vi "GatherBLTargets.vi"(11 "BL files folder path":path) -> (1 "BL Targets out":T1[](array[typedef]) {"n" min=0.02 max=0.5 step=0.01 format="%.2f"})   [LabVIEW 2016]
uses:
  BLTarget.ctl
  Globals/Constants_global.vi
panel:
  in  "BL Targets Manual":T1[](array[typedef])=[{"Code"="ASCE7 C", "TI Profile (FS)"=[[25.4, 12.0], [25.4, 14.0], [50.8, 13.0], [50.8, 11.0], [25.4, 12.0]], "n"=0.14}, {"Code"="B2", "TI Profile (FS)"=[[15.0, 25.5], [20.0, 24.3], [25.0, 23.5], [30.0, 22.9], [35.0, 22.3], [45.0, 21.5], [55.0, 20.9], [65.0, 20.4], [80.0, 19.7], [100.0, 19.0], [125.0, 18.2], [150.0, 17.6], [200.0, 16.5], [235.0, 15.8], [300.0, 14.7], [360.0, 13.9]], "n"=0.24}, {"Code"="C1", "TI Profile (FS)"=[[76.2, 10.28], [152.4, 8.46]], "n"=0.139}, {"Code"="C2", "TI Profile (FS)"=[[15.0, 16.0], [20.0, 15.6], [25.0, 15.2], [30.0, 14.9], [35.0, 14.7], [45.0, 14.2], [55.0, 13.9], [65.0, 13.5], [80.0, 13.0], [100.0, 12.5], [125.0, 11.9], [150.0, 11.4], [200.0, 10.5], [235.0, 10.0], [300.0, 9.2], [360.0, 8.6]], "n"=0.16000000000000003}, {"Code"="AB1", "TI Profile (FS)"=[[76.2, 29.33], [152.4, 22.56]], "n"=0.292}, {"Code"="D1", "TI Profile (FS)"=[[76.2, 12.115], [152.4, 11.19]], "n"=0.106}, {"Code"="Cat2", "TI Profile (FS)"=[[10.0, 20.7], [16.7, 19.6], [33.3, 18.3], [50.0, 17.6], [66.7, 17.1], [100.0, 16.2], [133.3, 15.6], [166.7, 15.1], [250.0, 14.0], [333.3, 13.1], [500.0, 11.7], [666.7, 10.8], [833.3, 9.8], [1000.0, 9.2], [1333.3, 8.2], [1666.7, 7.4], [3333.3, 7.4]], "n"=0.202}, {"Code"="Cat3", "TI Profile (FS)"=[[10.0, 27.1], [16.7, 27.1], [33.3, 23.9], [50.0, 22.5], [66.7, 21.5], [100.0, 20.3], [133.3, 19.5], [166.7, 18.8], [250.0, 17.6], [333.3, 16.6], [500.0, 15.0], [666.7, 13.9], [833.3, 12.9], [1000.0, 12.1], [1333.3, 10.8], [1666.7, 9.8], [3333.3, 9.8]], "n"=0.202}] {"n" min=0.02 max=0.5 step=0.01 format="%.2f"}
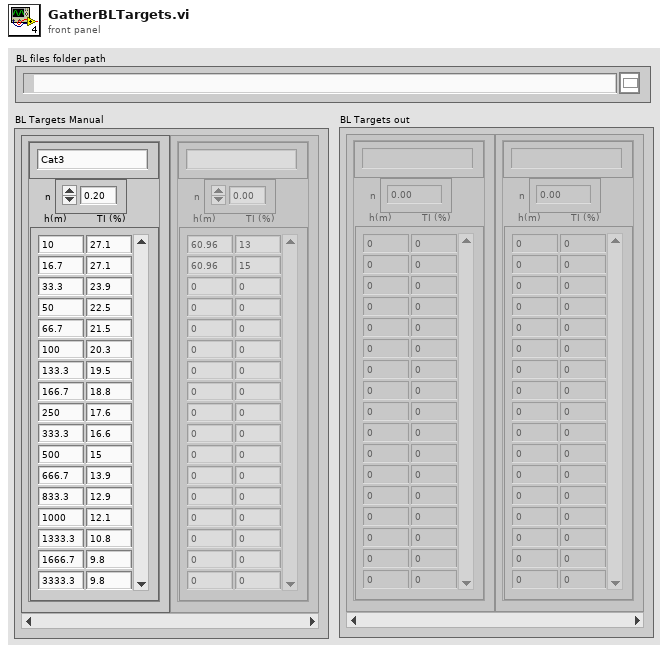
[diagram p1: front panel]
types:
  T1 = typedef "BLTarget.ctl" = cluster{"Code":string, "TI Profile (FS)":dbl[][], "n":dbl}
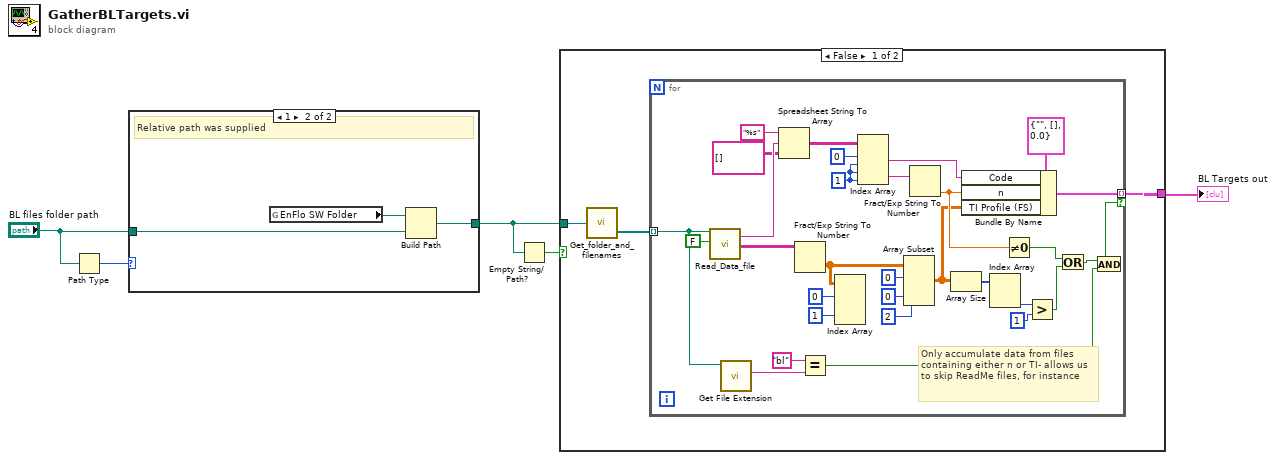
[diagram p0: block diagram]
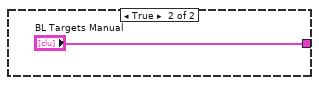
[diagram p3: hidden frame]
diagram:
  n1 = Path Type(1:"BL files folder path") -> (0:w3:i16)
  n2 = case shown="1" w3 {
    tunnel: "BL files folder path" -> [w6 w9]
    tunnel: [w6 w8] -> w1
    frame 0, Default {
      # "Absolute path- ready to go"
    }
    frame 1 {
      # "Relative path was supplied"
      n3 = global read "Constants_global.vi" "EnFlo SW Folder"() -> (w7:path)
      n4 = Build Path(base path=w7, name or relative path=w9) -> (appended path=w8:path)
    }
  }
  n5 = Empty String/Path?(string/path=w1) -> (empty?=w4:bool)
  n6 = case shown="False" w4 {
    tunnel: [w12 "BL Targets Manual"] -> w5
    tunnel: w1 -> [w11 _]
    frame False {
      n7 = call "Get_folder_and_filenames.vi"("file path (dialog if empty)"=w11) -> ("Files"=w10:path[])  [unwired: 1 out]
      n8 = for {
        tunnel: w10 -> [w18] mode=indexing
        tunnel: [w27] -> w12 mode=indexing if=w15
        w38 = 1 ("index (row)")
        # "Only accumulate data from files containing either n or TI- allows us to skip ReadMe files, for instance"
        n9 = call "Read_Data_file.vi"("Results file"=w18, "Delete First Rows?"=FALSE) -> ("String Before"=w43:string, "Channel Values Out"=w36:string[][])  [unwired: 7 in, 9 out]
        n10 = call <vilib>:"Get File Extension.vi"("file"=w18) -> ("lowercase file extension"=w17:string)  [unwired: 6 in, 4 out]
        n11 = Spreadsheet String To Array(format string="%s", spreadsheet string=w43, array type (2D Dbl)=string[][] []) -> (array=w40:string[][])  [unwired: 1 in]
        n12 = Fract/Exp String To Number(string=w36) -> (number=w33:dbl[][])  [unwired: 3 in, 1 out]
        n13 = Equal?(x="bl", y=w17) -> (x = y?=w14:bool)
        n14 = Index Array(array=w33, index (row) #1=0 ("index (row)"), index (row) #2=1 ("index (row)")) -> ()  [unwired: 2 in, 2 out]
        n15 = Index Array(array=w40, index (row) #1=0 ("index (row)"), index (col) #1=w38, index (row) #2=w38, index (col) #2=w38) -> (element #1=w28:string, element #2=w37:string)
        n16 = Array Subset(array=w33, index (row)=0 ("index"), index (col)=0 ("index"), length (col)=2 ("length")) -> (w25:dbl[][])  [unwired: 1 in]
        n17 = Fract/Exp String To Number(string=w37) -> (number=w26:dbl)  [unwired: 3 in, 1 out]
        n18 = Array Size(array=w25) -> (size(s)=w22:i32[])
        n19 = Bundle By Name(cluster=T1 {"Code"="", "TI Profile (FS)"=[], "n"=0.0} ("Cluster"), "Code"=w28, "n"=w26, "TI Profile (FS)"=w25) -> (w27:T1)
        n20 = Index Array(array=w22) -> (element #2=w21:i32)  [unwired: 2 in, 1 out]
        n21 = Not Equal To 0?(x=w26) -> (x != 0?=w24:bool)
        n22 = Greater?(x=w21, y=1) -> (0:w19:bool)
        n23 = Or(x=w24, y=w19) -> (x .or. y?=w23:bool)
        n24 = And(x=w23, y=w14) -> (x .and. y?=w15:bool)
      }
    }
    frame True {
    }
  }
  "BL Targets out" <- w5
